vi "Test Open Read Close MP3.vi"(8 "error in (no error)":errorcluster) -> (0 "error out":errorcluster, 3 "Pass?":bool)   [LabVIEW 2020]
uses:
  f10b0684-7096-4b01-9a3f-e3a173c30d84.vi
  e2b84ce0-42ce-4834-8995-1adf876162a5.vi
  G-Audio/Private/Get Basic Audio File Info.vi
  G-Audio/Private/Result To Error.vi
  f10b0684-7096-4b01-9a3f-e3a173c30d84.vi/779dfdfd-1b42-4cf4-8001-66d3dd167625.vi
  f10b0684-7096-4b01-9a3f-e3a173c30d84.vi/55d550d4-9624-414e-aebd-6e02b5081896.vi
  f10b0684-7096-4b01-9a3f-e3a173c30d84.vi/779dfdfd-1b42-4cf4-8001-66d3dd167625.vi/a9d2058a-38f9-4c88-a1a9-9bf864ebbde5.vi
  f10b0684-7096-4b01-9a3f-e3a173c30d84.vi/55d550d4-9624-414e-aebd-6e02b5081896.vi/4b7b629c-2e91-4160-9820-a26af8f6e677.vi
  f10b0684-7096-4b01-9a3f-e3a173c30d84.vi/55d550d4-9624-414e-aebd-6e02b5081896.vi/e7c4a249-ce38-42b4-8985-5fdb76b4ebfc.vi
  <vilib>/sound2/lvsound2.llb/Sound File Read Open.vi
  <vilib>/sound2/lvsound2.llb/Sound File Info (refnum).vi
  <vilib>/sound2/lvsound2.llb/Sound File Read (I16).vi
  <vilib>/Utility/Data Type/Get Numeric Information.vi
  <vilib>/Utility/error.llb/Error Cluster From Error Code.vi
  G-Audio/G-Audio.lvlib
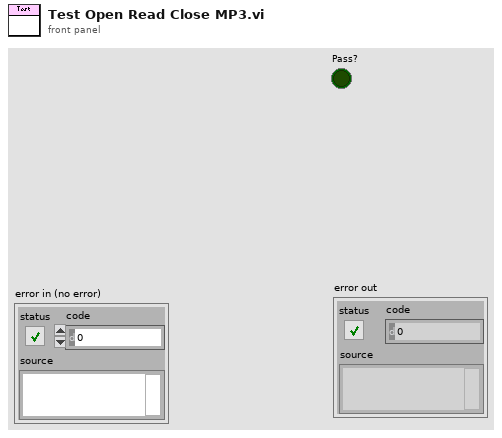
[diagram p1: front panel]
types:
  T1 = typedef "G-Audio.lvlib/Audio File Info.ctl" = cluster{"Sample Rate (Hz)":u32, "Channels":u32, "Bit Depth":u32}
  T2 = typedef "Sound File Refnum.ctl" = refnum<file>
  T3 = typedef "Sound Data Format.ctl" = cluster{"sample rate (S/s)":dbl, "number of channels":i32, "bits per sample":i32}
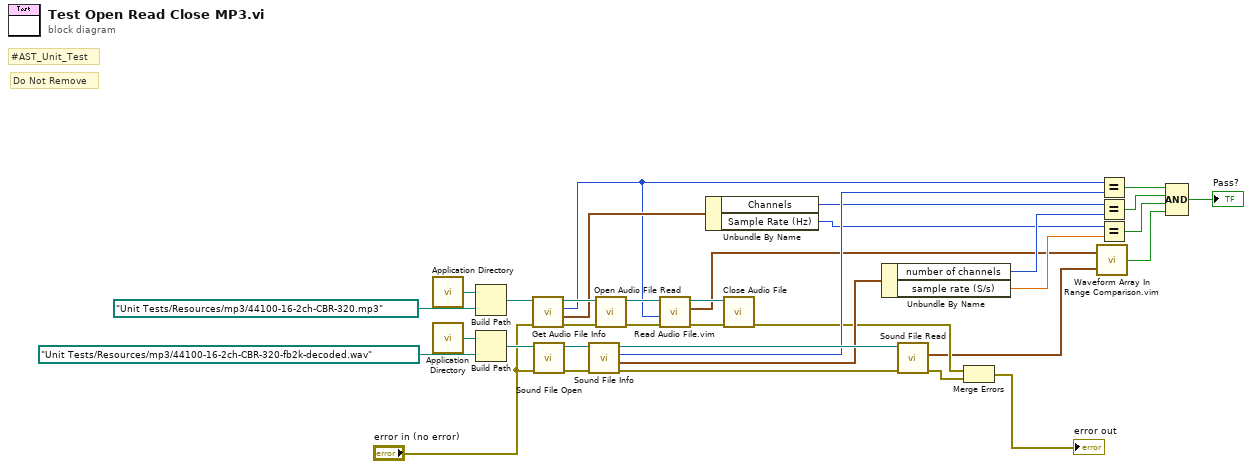
[diagram p0: block diagram]
diagram:
  # "Do Not Remove"
  # "#AST_Unit_Test"
  n1 = call <vilib>:"Application Directory.vi"() -> ("Application Directory"=w3:path)
  n2 = call <vilib>:"Application Directory.vi"() -> ("Application Directory"=w35:path)
  n3 = Build Path(base path=w3, name or relative path=path "Unit Tests/Resources/mp3/44100-16-2ch-CBR-320.mp3" ("Path")) -> (appended path=w1:path)
  n4 = Build Path(base path=w35, name or relative path=path "Unit Tests/Resources/mp3/44100-16-2ch-CBR-320-fb2k-decoded.wav" ("Path")) -> (appended path=w34:path)
  n5 = call "Get Audio File Info.vi"("error in (no error)"="error in (no error)", "Path In"=w1) -> ("error out"=w12:errorcluster, "Audio File Info"=w16:T1, "Sample Length"=w4:u64, "Path Out"=w18:path)  [unwired: 6 in]
  n6 = call-poly <vilib>:"Sound File Open.vi"("error in (no error)"="error in (no error)", "path"=w34) -> ("error out"=w23:errorcluster, "sound file refnum"=w32:T2)  [unwired: 8 in]
  n7 = call-poly <vilib>:"Sound File Info.vi"("error in (no error)"=w23, "sound file refnum"=w32) -> ("error out"=w22:errorcluster, "sound format"=w27:T3, "total number of samples/ch"=w28:u32, "sound file refnum out"=w31:T2)  [unwired: 6 in]
  n8 = call "Open Audio File Read.vi"("error in (no error)"=w12, "Path"=w18) -> ("error out"=w11:errorcluster, "Audio File Refnum"=w17:refnum<file>)  [unwired: 8 in]
  n9 = call "Read Audio File.vim"("error in (no error)"=w11, "Samples To Read"=w4, "Audio File Refnum In"=w17) -> ("error out"=w9:errorcluster, "Audio Data"=w6:waveform(i16)[], "Audio File Refnum Out"=w10:refnum<file>)  [unwired: 4 in, 2 out]
  n10 = Unbundle By Name(w16) -> ("Channels"=w15:u32, "Sample Rate (Hz)"=w14:u32)
  n11 = call "Close Audio File.vi"("error in (no error)"=w9, "Audio File Refnum In"=w10) -> ("error out"=w8:errorcluster)  [unwired: 9 in]
  n12 = Unbundle By Name(w27) -> ("number of channels"=w26:i32, "sample rate (S/s)"=w19:dbl)
  n13 = call-poly <vilib>:"Sound File Read.vi"("error in (no error)"=w22, "sound file refnum"=w31) -> ("error out"=w21:errorcluster, "data"=w7:waveform(i16)[])  [unwired: 5 in, 3 out]
  n14 = Merge Errors(w8, w21) -> (→"error out":errorcluster)
  n15 = call "Waveform Array In Range Comparison.vim"("Expected Value"=w7, "Resulting Value"=w6) -> ("Comparison Result"=w5:bool)
  n16 = Equal?(x=w4, y=w28) -> (x = y?=w30:bool)
  n17 = Equal?(x=w15, y=w26) -> (x = y?=w25:bool)
  n18 = Equal?(x=w14, y=w19) -> (x = y?=w24:bool)
  n19 = Compound Arithmetic op=AND(w30, w25, w24, w5) -> (→"Pass?":bool)
